vi "To Field Centric.vi"(10 "IMU Value (offset)":dbl, 11 "Translation Joystick":cluster{dbl, dbl}) -> (1 "IMU (radians)":dbl, 2 "Robot Centric Vector":cluster{dbl, dbl}, 3 "Joystick (Field Centric) Polar Vector":cluster{dbl, dbl})   [LabVIEW 2020]
uses:
  <vilib>/Analysis/coordinate.llb/Angle Units.ctl
  <vilib>/Analysis/coordinate.llb/Angle Range (Degree).ctl
  <vilib>/Analysis/coordinate.llb/Wrap Angle (scalar).vi
  <vilib>/Analysis/NI_AAL_Angle.lvlib
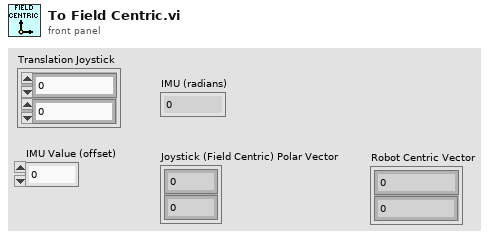
[diagram p1: front panel]
types:
  T1 = typedef "NI_AAL_Angle.lvlib/Angle Range (Degree).ctl" = u16
  T2 = typedef "NI_AAL_Angle.lvlib/Angle Units.ctl" = i32
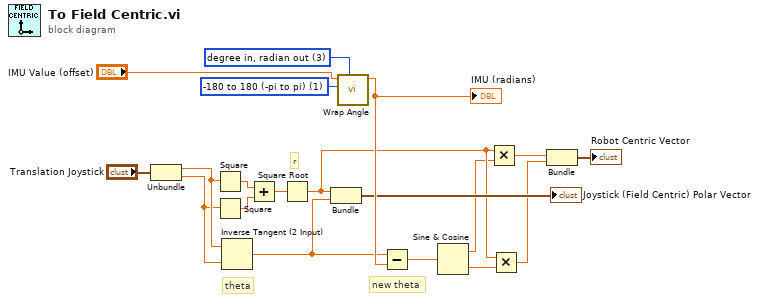
[diagram p0: block diagram]
diagram:
  w18 = T1 1 items=["none", "-180 to 180 (-pi to pi)", "0 to 360 (0 to 2pi)"] ("angle range")
  w19 = T2 3 items=["radian in, radian out", "radian in, degree out", "degree in, degree out", "degree in, radian out"] ("angle units")
  # "new theta"
  # "theta"
  # "r"
  n1 = Unbundle("Translation Joystick") -> (w2:dbl, w1:dbl)
  n2 = Square(x=w2) -> (x^2=w16:dbl)
  n3 = Square(x=w1) -> (x^2=w15:dbl)
  n4 = Inverse Tangent (2 Input)(1:w1, 2:w2) -> (0:w12:dbl)
  n5 = Add(x=w16, y=w15) -> (x+y=w14:dbl)
  n6 = Square Root(x=w14) -> (sqrt(x)=w10:dbl)
  n7 = Bundle(w10, w12) -> (→"Joystick (Field Centric) Polar Vector":cluster{dbl, dbl})  [unwired: 1 in]
  n8 = call-poly <vilib>:"Wrap Angle.vi"("angle units"=w19, "angle range"=w18, "angle in"="IMU Value (offset)") -> ("angle out"=w13:dbl)  [unwired: 7 in, 1 out]
  "IMU (radians)" <- w13
  n9 = Subtract(x=w12, y=w13) -> (x-y=w6:dbl)
  n10 = Sine & Cosine(0:w6) -> (1:w4:dbl, 2:w5:dbl)
  n11 = Multiply(x=w10, y=w4) -> (x*y=w9:dbl)
  n12 = Multiply(x=w10, y=w5) -> (x*y=w8:dbl)
  n13 = Bundle(w9, w8) -> (→"Robot Centric Vector":cluster{dbl, dbl})  [unwired: 1 in]
